vi "Iterative Operations.vi"(8 "error in":errorcluster, 9 "Input Paths":T1={"Golden Template (Source) - (make relative)"=path "E:/Documents/Projects/SPIAPI/Github/SPIFramework/IONode", "Destination Generated Code (make relative)"=path "E:/Documents/Projects/SPIAPI/Github/SPIFramework/Test", "LabVIEW Project to Script"=path "E:/Documents/Projects/SPIAPI/Github/SPIFramework/Test/Test.lvproj", "Placement VI"=path "E:/Documents/Projects/SPIAPI/Github/SPIFramework/Test/TestVI.VI"}, 10 "Current Bus Number":i32, 11 "Queue in":refnum<queue>) -> (0 "error out":errorcluster, 1 "Current Status":string, 2 "Next State":T2, 3 "Queue out":refnum<queue>)   [LabVIEW 2014, in "SPI Engine Scripting.lvlib"]
doc: "Checks for errors, manages the Scripting Log and dequeues the next states in the scripting process."
uses:
  SPI Engine Scripting.lvlib
  Scripting States.ctl
  Controls/Input Paths.ctl
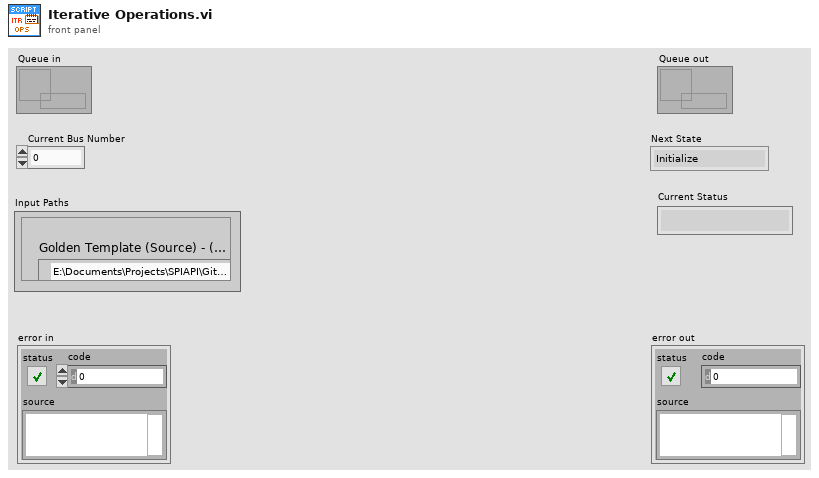
[diagram p1: front panel]
types:
  T1 = typedef "SPI Engine Scripting.lvlib/Input Paths.ctl" = cluster{"Golden Template (Source) - (make relative)":path, "Destination Generated Code (make relative)":path, "LabVIEW Project to Script":path, "Placement VI":path}
  T2 = typedef "Scripting States.ctl" = enum16{"Initialize", "Copy Template Bus Directory", "Modify Dequeue Commands", "Modify Enqueue Data", "Create FPGA VI", "Create Project FIFOs", "Create FPGA Data Nodes", "Place FPGA Data Nodes", "Update Node Count in Engine", "Expand FIFO Type Def", "Populate FIFO Names in Engine", "Modify I/O Pin Names", "Modify I/O Pin Enable", "Replace DLU", "Add Engine to Project", "Place SPI Engine", "Scripting Complete Check", "End"}
  T3 = enum16{"open", "replace", "create", "open or create", "replace or create", "replace or create with confirmation"}
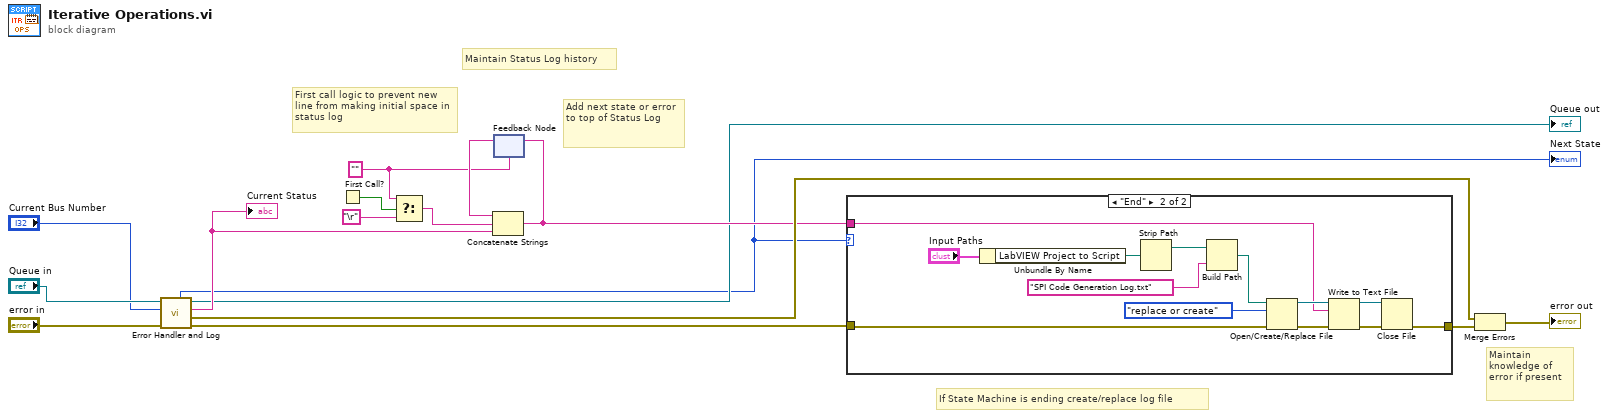
[diagram p0: block diagram]
diagram:
  w7 = ""
  # "Add next state or error to top of Status Log"
  # "Maintain Status Log history"
  # "First call logic to prevent new line from making initial space in status log"
  # "If State Machine is ending create/replace log file"
  # "Maintain knowledge of error if present"
  n1 = call "Error Handler and Log.vi"("error in (no error)"="error in", "Current Bus Number"="Current Bus Number", "Queue in"="Queue in") -> ("error out"=w3:errorcluster, "error out (maintain error)"=w12:errorcluster, "Current Status"=w5:string, "Queue out"=→"Queue out":refnum<queue>, "Next State"=w1:T2)  [unwired: 4 in]
  "Next State" <- w1
  "Current Status" <- w5
  n2 = First Call?() -> (First Call?: T/F=w8:bool)
  n3 = Select(t=w7, s=w8, f="\r") -> (s? t:f=w9:string)
  n4 = feedback #1(w7) -> (w11:string)
  n5 = Concatenate Strings(w11, w9, w5) -> (w6:string)
  n6 = feedback-in #1(w6) -> ()
  n7 = case shown="\"End\"" w1 {
    tunnel: [w17 w28] -> w4
    tunnel: w3 -> [w17 w23]
    tunnel: w6 -> [_ w21]
    frame Default {
    }
    frame "End" {
      n8 = Unbundle By Name("Input Paths") -> ("LabVIEW Project to Script"=w19:path)
      n9 = Strip Path(path=w19) -> (stripped path=w18:path)  [unwired: 1 out]
      n10 = Build Path(base path=w18, name or relative path="SPI Code Generation Log.txt") -> (appended path=w26:path)
      n11 = Open/Create/Replace File(file path (use dialog)=w26, error in=w23, operation (0:open)=T3."replace or create") -> (refnum out=w22:refnum<file>, error out=w24:errorcluster)  [unwired: 3 in, 1 out]
      n12 = Write to Text File(file (use dialog)=w22, text=w21, error in=w24) -> (refnum out=w29:refnum<file>, error out=w30:errorcluster)  [unwired: 1 in, 1 out]
      n13 = Close File(refnum=w29, error in=w30) -> (error out=w28:errorcluster)  [unwired: 1 out]
    }
  }
  n14 = Merge Errors(w12, w4) -> (→"error out":errorcluster)
